vi "MWriteRS232_2.vi"(0 "PORT PUMP3":i32=8, 1 "PORT PUMP2":i32=7, 2 "PORT PUMP1":i32=6, 3 "PORT LAUDA":i32=1, 5 "enable3":i32, 6 "enable4":i32, 7 "enable2":i32, 8 "P3":dbl, 9 "P2":dbl, 10 "P1":dbl, 11 "LAUDA":dbl=22.0) -> ()   [LabVIEW 2017]
uses:
  BERTTA.dll
panel:
  in  "dev4":i32=2
  in  "dev3":i32=2
  in  "dev2":i32=3
  in  "dev1":i32=1
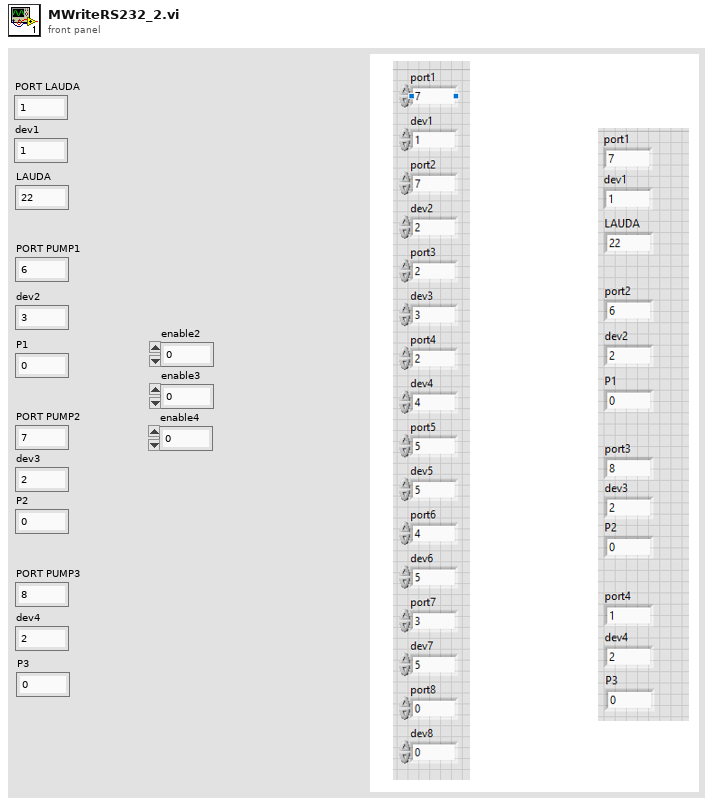
[diagram p1: front panel]
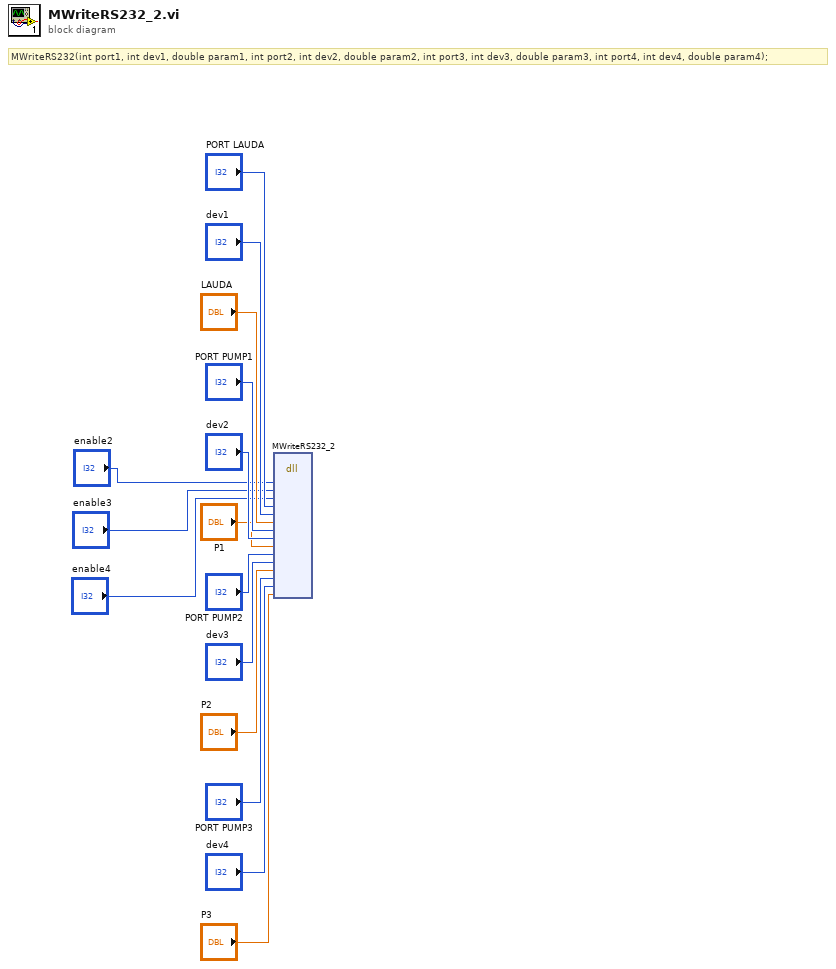
[diagram p0: block diagram]
diagram:
  # "MWriteRS232(int port1, int dev1, double param1, int port2, int dev2, double param2, int port3, int dev3, double param3, int port4, int dev4, double param4);"
  n1 = dll-call lib="C:/Users/shresplab/OneDrive - Kemira Oyj/Documents/GitHub/Bertta/BERTTA/x64/Debug/BERTTA.dll" fn="MWriteRS232_2"("enable2"="enable2", "enable3"="enable3", "enable4"="enable4", "port1"="PORT LAUDA", "dev1"="dev1", "param1"="LAUDA", "port2"="PORT PUMP1", "dev2"="dev2", "param2"="P1", "port3"="PORT PUMP2", "dev3"="dev3", "param3"="P2", "port4"="PORT PUMP3", "dev4"="dev4", "param4"="P3") -> ()  [unwired: 19 in, 2 out]
